vi "TDC_setLftParams.vi"(8 "Error In":errorcluster, 9 "Bin width [ps]":i32=2, 10 "Bin Count":i32=100) -> (0 "Error Out":errorcluster)   [LabVIEW 2011]
uses:
  tdcbase.dll
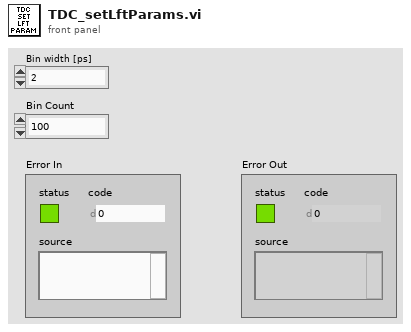
[diagram p1: front panel]
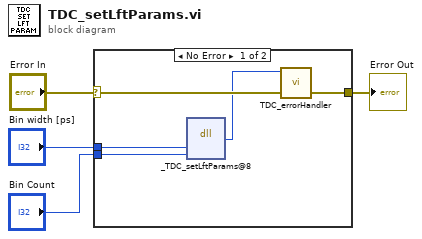
[diagram p0: block diagram]
diagram:
  n1 = case shown="No Error" "Error In" {
    selector: "Error In" -> [w8 w10]
    tunnel: [w7 w10] -> w3
    tunnel: "Bin width [ps]" -> [w9 _]
    tunnel: "Bin Count" -> [w6 _]
    frame No Error {
      n2 = dll-call lib="X:/tdcbase.dll" fn="_TDC_setLftParams@8"("binWidth"=w9, "binCount"=w6) -> ("return type"=w5:i32)  [unwired: 5 in, 2 out]
      n3 = call "TDC_errorHandler.vi"("Error In"=w8, "TDC Return Code"=w5) -> ("Error Out"=w7:errorcluster)  [unwired: 9 in]
    }
    frame Error {
    }
  }
  "Error Out" <- w3
